vi "Recursive_6733_Init.vi"(4 "Error In":errorcluster, 5 "task in":refnum<k21>, 6 "Counter":i32, 7 "Stop and Clear?":bool) -> (0 "error out":errorcluster={"status"=TRUE, "code"=-89125, "source"="6733_88_write_waveform_2014.11.21.vi<append>\n<B>Source Device: </B>6733_Red_88\n<B>Destination Device: </B>6733_Red_87\n\n<B>Task Name: </B>Red MOT 88 Wfm"}, 2 "task out":refnum<k21>)   [LabVIEW 2016]
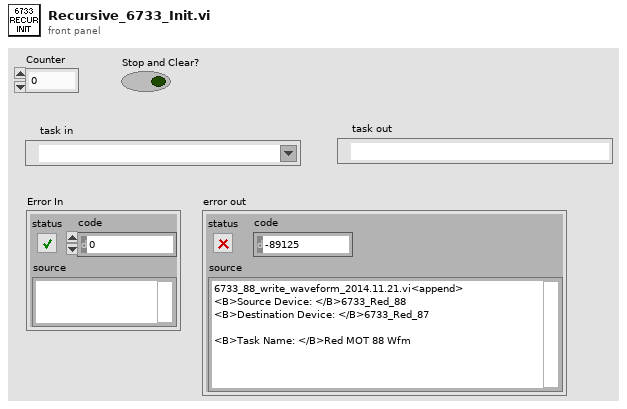
[diagram p1: front panel]
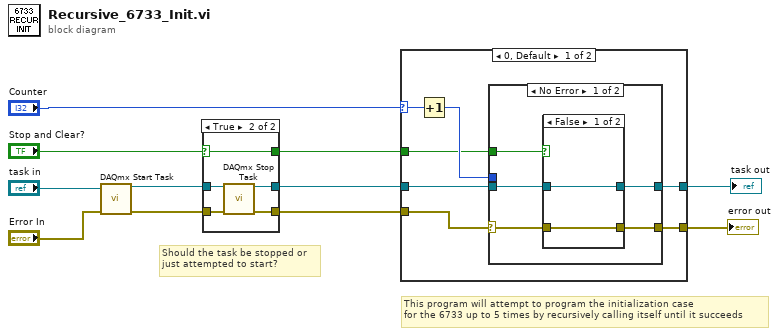
[diagram p0: block diagram]
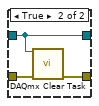
[diagram p3: hidden frame]
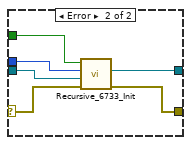
[diagram p4: hidden frame]
diagram:
  # "Should the task be stopped or\njust attempted to start?"
  # "This program will attempt to program the initialization case\nfor the 6733 up to 5 times by recursively calling itself until it succeeds"
  n1 = call <vilib>:"DAQmx Start Task.vi"("task/channels in"="task in", "error in"="Error In") -> ("task out"=w10:refnum<k21>, "error out"=w8:errorcluster)  [unwired: 12 in]
  n2 = case shown="True" "Stop and Clear?" {
    selector: "Stop and Clear?" -> [w12 w15]
    tunnel: w10 -> [w14 w19]
    tunnel: w8 -> [w13 w18]
    tunnel: [w13 w17] -> w7
    tunnel: [w14 w16] -> w6
    tunnel: [w12 w15] -> w1
    frame False {
    }
    frame True {
      n3 = call <vilib>:"DAQmx Stop Task.vi"("task/channels in"=w19, "error in"=w18) -> ("task out"=w16:refnum<k21>, "error out"=w17:errorcluster)  [unwired: 12 in]
    }
  }
  n4 = case shown="0, Default" "Counter" {
    selector: "Counter" -> [w22 _]
    tunnel: w7 -> [w26 w44]
    tunnel: w6 -> [w25 w43]
    tunnel: [w24 w44] -> w3
    tunnel: [w23 w43] -> w5
    tunnel: w1 -> [w20 _]
    frame 0, Default {
      n5 = Increment(x=w22) -> (x+1=w21:i32)
      n6 = case shown="No Error" w26 {
        selector: w26 -> [w31 w42]
        tunnel: w25 -> [w30 w39]
        tunnel: [w29 w41] -> w24
        tunnel: [w27 w40] -> w23
        tunnel: w21 -> [_ w38]
        tunnel: w20 -> [w28 w37]
        frame No Error {
          n7 = case shown="False" w28 {
            tunnel: w31 -> [w32 w36]
            tunnel: w30 -> [w33 w34]
            tunnel: [w32 w35] -> w29
            tunnel: [w33 w34] -> w27
            frame False {
            }
            frame True {
              n8 = call <vilib>:"DAQmx Clear Task.vi"("task in"=w34, "error in"=w36) -> ("error out"=w35:errorcluster)  [unwired: 13 in]
            }
          }
        }
        frame Error {
          n9 = call "Recursive_6733_Init.vi"("Error In"=w42, "task in"=w39, "Counter"=w38, "Stop and Clear?"=w37) -> ("error out"=w41:errorcluster, "task out"=w40:refnum<k21>)  [unwired: 2 in]
        }
      }
    }
    frame 5 {
    }
  }
  "error out" <- w3
  "task out" <- w5
